vi "test_BuildEvalStr_FP_Equal.vi"(8 "error in (no error)":errorcluster, 11 "TestCase in":refnum<class "Build Eval Str Test Case.lvclass">) -> (0 "error out":errorcluster, 3 "TestCase out":refnum<class "Build Eval Str Test Case.lvclass">)   [LabVIEW 2018, in "Build Eval Str Test Case.lvclass"]
uses:
  Build Eval Str Test Case.lvclass
  Plugins/Utility/Test Classes/Floating Point/Equal/FP Equal.lvclass
  C:/Users/UKHornP/Documents/Work/Projects/Assert_API/Plugins/Utility/Test Classes/Floating Point/Floating Point.lvclass
  C:/Users/UKHornP/Documents/Work/Projects/Assert_API/Plugins/Utility/Test Classes/Test.lvclass
  Plugins/Utility/Test Classes/Floating Point/Floating Point.lvclass/Floating Point.ctl
  Plugins/Utility/Test Classes/Test Class String IDs.vi
  <vilib>/addons/_JKI Toolkits/VI Tester/TestCase.llb/TestCase.lvclass
  Plugins/Utility/Test Classes/Test.lvclass
  Plugins/Utility/Test Classes/Floating Point/Floating Point.lvclass
  C:/Program Files (x86)/National Instruments/LabVIEW 2018/vi.lib/addons/_JKI Toolkits/VI Tester/TestCase.llb/TestCase.lvclass
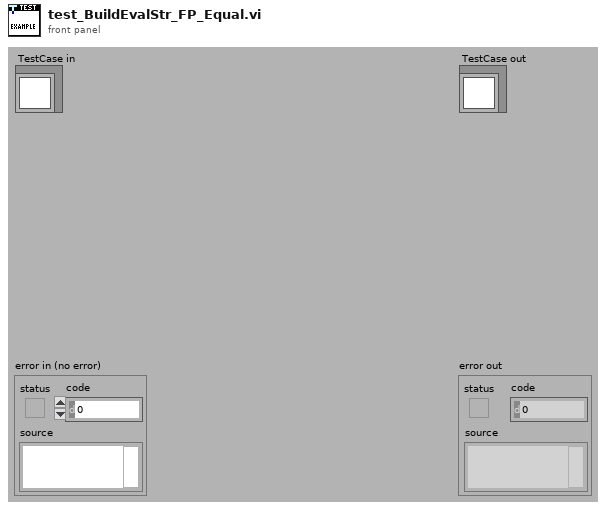
[diagram p1: front panel]
types:
  T1 = cluster{"Comparison Value 1":string, "Comparison Value 2":string, "Invert Result":string, "Assert VI Name":string, "Data Type":string, "Builder User Name":string, "Build Timestamp":string, "Failure Action":string, "Comment":string, "Assert Name":string, "Description":string, "Evaluation String":string}
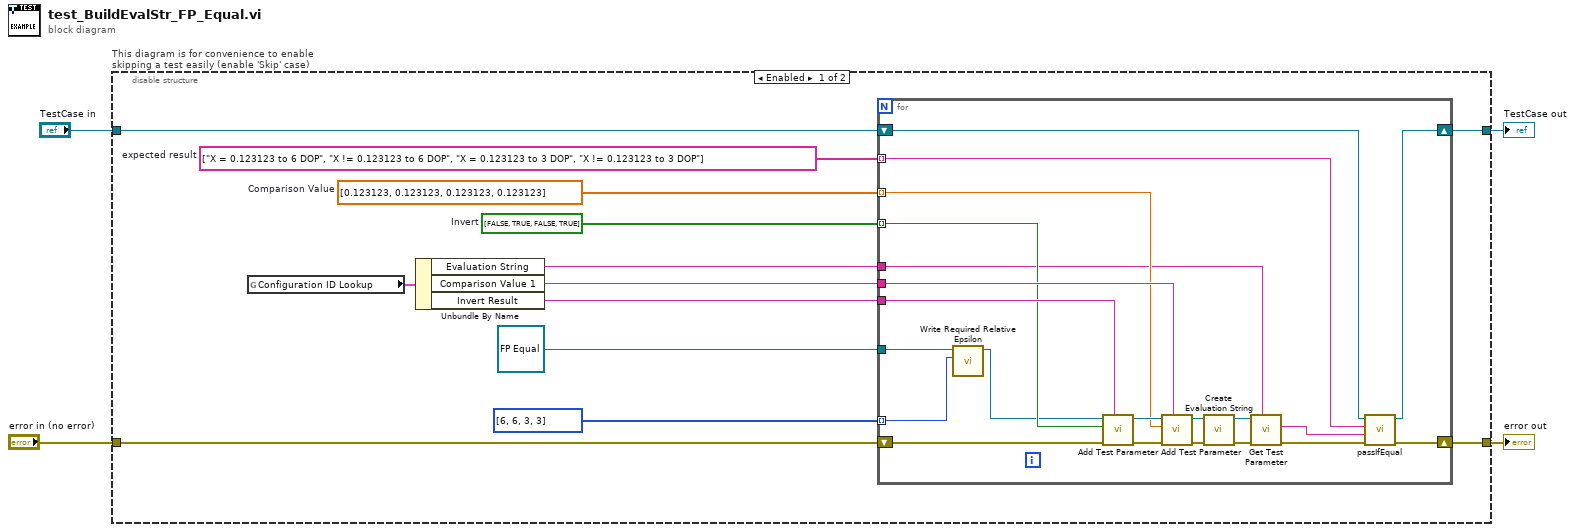
[diagram p0: block diagram]
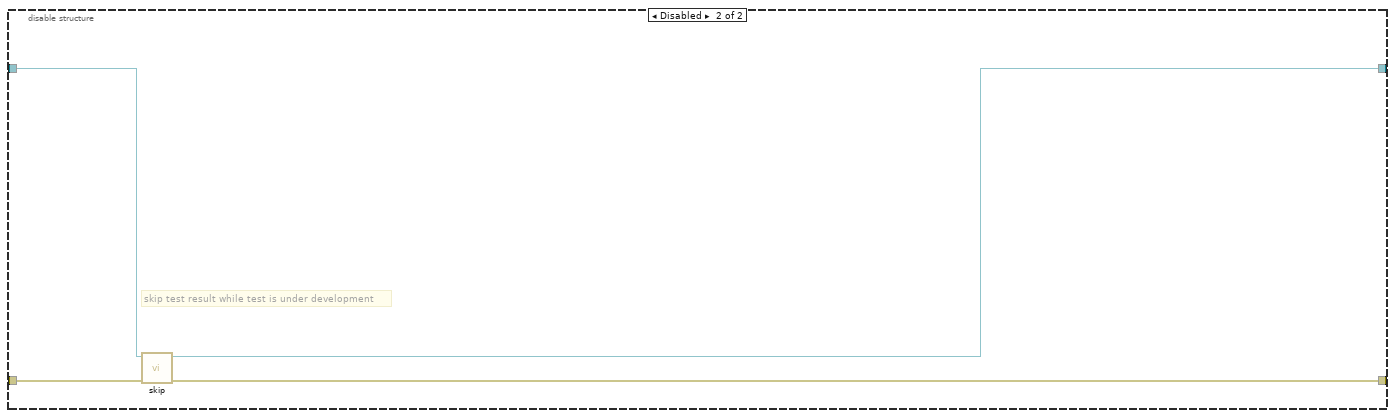
[diagram p2: hidden frame]
diagram:
  n1 = disable-structure "This diagram is for convenience to enable skipping a test easily (enable 'Skip' case)" shown="Enabled" {
    disable-tunnel: "TestCase in" -> [w16 w42]
    disable-tunnel: [w15 w40] -> w1
    disable-tunnel: [w14 w41] -> w3
    disable-tunnel: "error in (no error)" -> [w7 w39]
    frame Enabled {
      w8 = dbl[] [0.123123, 0.123123, 0.123123, 0.123123]  # Comparison Value
      w9 = bool[] [FALSE, TRUE, FALSE, TRUE]  # Invert
      w17 = string[] ["X = 0.123123 to 6 DOP", "X != 0.123123 to 6 DOP", "X = 0.123123 to 3 DOP", "X != 0.123123 to 3 DOP"]  # expected result
      n2 = global read "Test Class String IDs.vi" "Configuration ID Lookup"() -> (w12:T1)
      n3 = Unbundle By Name(w12) -> ("Evaluation String"=w6:string, "Comparison Value 1"=w10:string, "Invert Result"=w11:string)
      n4 = for {
        tunnel: w17 -> [w38] mode=indexing
        tunnel: refnum<class "FP Equal.lvclass"> refnum ("FP Equal.lvclass") -> [w20]
        tunnel: w11 -> [w34]
        tunnel: w10 -> [w33]
        tunnel: w9 -> [w31] mode=indexing
        tunnel: w8 -> [w30] mode=indexing
        tunnel: w6 -> [w22]
        shift-right: [w36] -> w15
        shift-left: w16 -> [w37]
        shift-right: [w35] -> w14
        shift-left: w7 -> [w29]
        tunnel: u8[] [6, 6, 3, 3] ("Required Digits of Precision") -> [w18] mode=indexing
        n5 = call "Write Required Relative Epsilon.vi"("Required Relative Epsilon"=w18, "Floating Point in"=w20) -> ("Floating Point out"=w19:refnum<class "FP Equal.lvclass">)  [unwired: 9 in]
        n6 = call-dynamic "Add Test Parameter.vi"("Data Value ID"=w34, "error in (no error)"=w29, "Data Value"=w31, "Test in"=w19) -> ("error out"=w28:errorcluster, "Test out"=w32:refnum<class "FP Equal.lvclass">)  [unwired: 5 in, 1 out]
        n7 = call-dynamic "Add Test Parameter.vi"("Data Value ID"=w33, "error in (no error)"=w28, "Data Value"=w30, "Test in"=w32) -> ("error out"=w26:errorcluster, "Test out"=w27:refnum<class "FP Equal.lvclass">)  [unwired: 5 in, 1 out]
        n8 = call-dynamic "Create Evaluation String.vi"("error in (no error)"=w26, "FP Equal in"=w27) -> ("error out"=w25:errorcluster, "FP Equal out"=w23:refnum<class "FP Equal.lvclass">)  [unwired: 8 in]
        n9 = call "Get Test Parameter.vi"("Data Value ID"=w22, "error in (no error)"=w25, "Test in"=w23) -> ("error out"=w24:errorcluster, "Test Parameter"=w21:string)  [unwired: 6 in, 1 out]
        n10 = call-dynamic "passIfEqual.vi"("error in (no error)"=w24, "y"=w21, "x"=w38, "TestCase in"=w37) -> ("error out"=w35:errorcluster, "TestCase out"=w36:refnum<class "Build Eval Str Test Case.lvclass">)  [unwired: 6 in]
      }
    }
    frame Disabled {
      # "skip test result while test is under development"
      n11 = call <vilib>:"skip.vi"("error in (no error)"=w39, "TestCase in"=w42) -> ("error out"=w41:errorcluster, "TestCase out"=w40:refnum<class "Build Eval Str Test Case.lvclass">)  [unwired: 8 in]
    }
  }
  "error out" <- w3
  "TestCase out" <- w1
